vi "RUSHShoot.vi"(1 "In Cluster":T2) -> (0 "Out Cluster":T1)   [LabVIEW 2012]
panel:
  in  "Highest POT pos":dbl=5.0
  in  "Lowest POT pos":dbl
  in  "ShootPOTToPowConst":dbl=0.2
  in  "Vision Speed Const":dbl=0.75
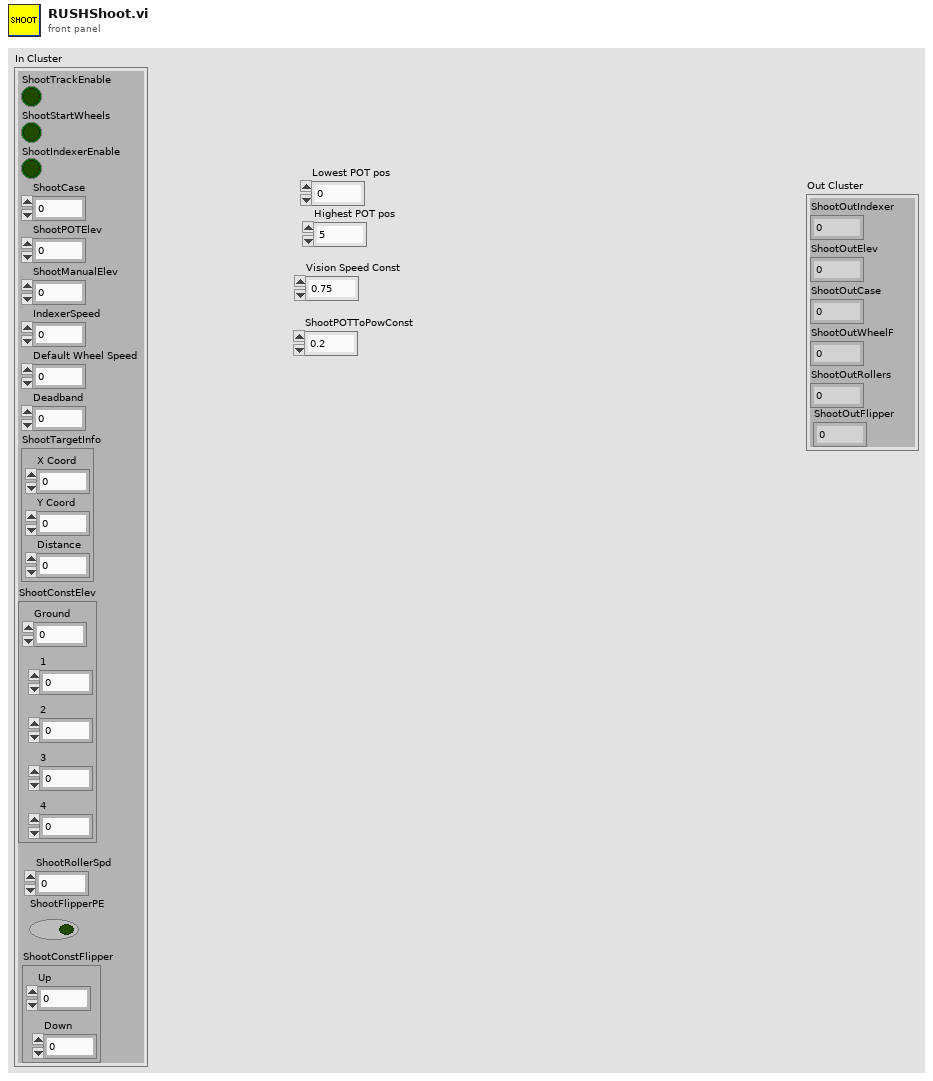
[diagram p1: front panel]
types:
  T1 = cluster{"ShootOutIndexer":dbl, "ShootOutElev":dbl, "ShootOutCase":dbl, "ShootOutWheelF":dbl, "ShootOutRollers":dbl, "ShootOutFlipper":dbl}
  T2 = cluster{"ShootTrackEnable":bool, "ShootStartWheels":bool, "ShootIndexerEnable":bool, "ShootCase":dbl, "ShootPOTElev":dbl, "ShootManualElev":dbl, "IndexerSpeed":dbl, "Default Wheel Speed":dbl, "Deadband":dbl, "ShootTargetInfo":cluster{"X Coord":dbl, "Y Coord":dbl, "Distance":dbl}, "ShootConstElev":cluster{"1":dbl, "2":dbl, "3":dbl, "4":dbl, "Ground":dbl}, "ShootRollerSpd":dbl, "ShootFlipperPE":bool, "ShootConstFlipper":cluster{"Down":dbl, "Up":dbl}}
  T3 = cluster{"X Coord":dbl, "Y Coord":dbl, "Distance":dbl}
  T4 = cluster{"1":dbl, "2":dbl, "3":dbl, "4":dbl, "Ground":dbl}
  T5 = cluster{"f":dbl, "y":dbl, "f":dbl, "f":dbl, "f":dbl, "Down":dbl}
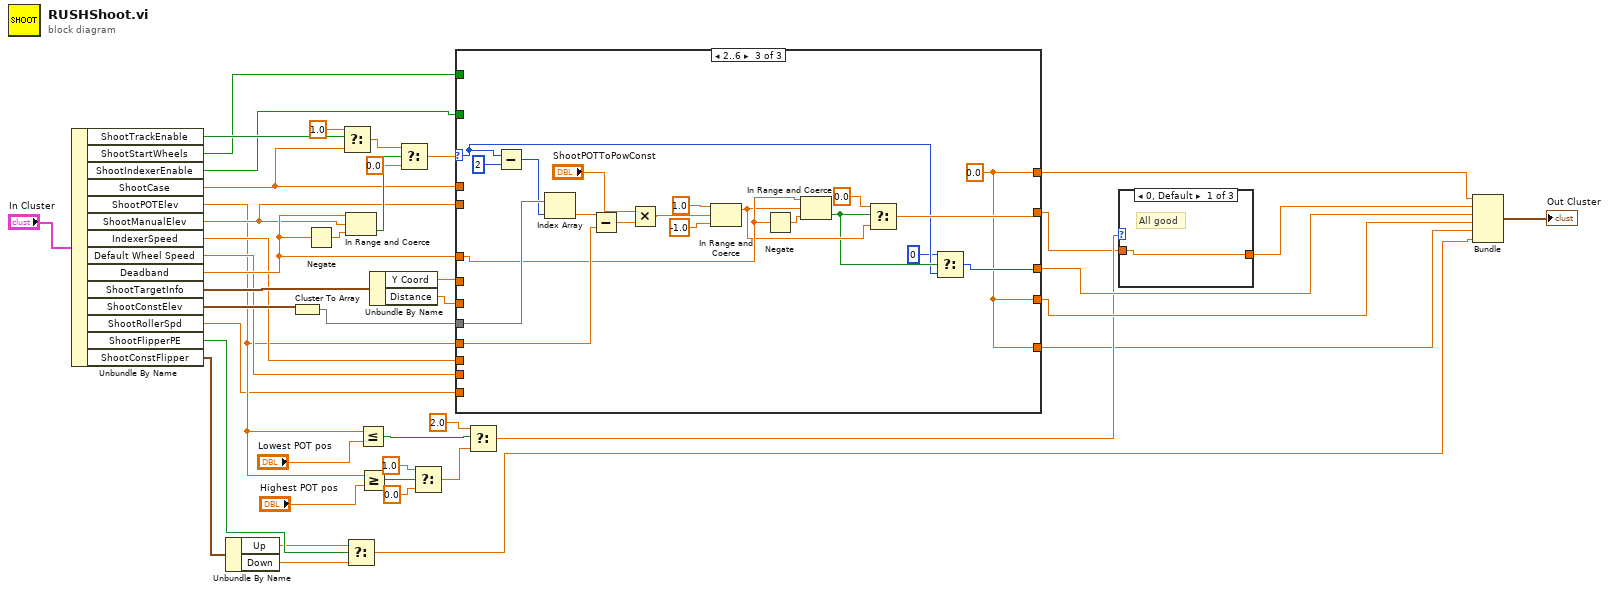
[diagram p0: block diagram]
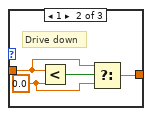
[diagram p2: hidden frame]
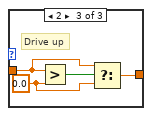
[diagram p3: hidden frame]
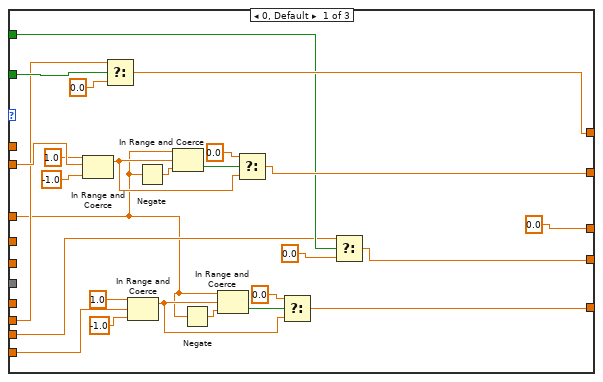
[diagram p4: hidden frame]
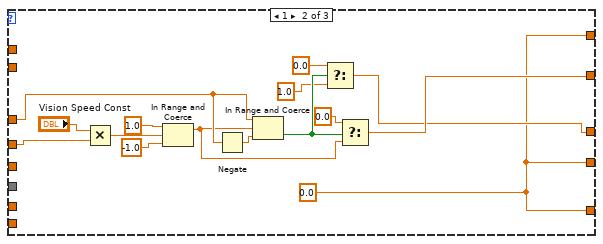
[diagram p5: hidden frame]
diagram:
  n1 = Unbundle By Name("In Cluster") -> ("ShootTrackEnable"=w42:bool, "ShootStartWheels"=w30:bool, "ShootIndexerEnable"=w29:bool, "ShootCase"=w31:dbl, "ShootPOTElev"=w18:dbl, "ShootManualElev"=w28:dbl, "IndexerSpeed"=w21:dbl, "Default Wheel Speed"=w20:dbl, "Deadband"=w32:dbl, "ShootTargetInfo"=w35:T3, "ShootConstElev"=w27:T4, "ShootRollerSpd"=w7:dbl, "ShootFlipperPE"=w3:bool, "ShootConstFlipper"=w4:cluster{"Down":dbl, "Up":dbl})
  n2 = Unbundle By Name(w4) -> ("Up"=w2:dbl, "Down"=w5:dbl)
  n3 = Cluster To Array(cluster=w27) -> (array=w26:dbl[])
  n4 = Negate(x=w32) -> (-x=w39:dbl)
  n5 = Select(t=1.0, s=w42, f=w31) -> (s? t:f=w40:dbl)
  n6 = In Range and Coerce(upper limit=w32, x=w28, lower limit=w39) -> (In Range?=w38:bool)  [unwired: 1 out]
  n7 = Select(t=w2, s=w3, f=w5) -> (s? t:f=w1:dbl)
  n8 = Less Or Equal?(x=w18, y="Lowest POT pos") -> (x <= y?=w12:bool)
  n9 = Greater Or Equal?(x=w18, y="Highest POT pos") -> (x >= y?=w16:bool)
  n10 = Unbundle By Name(w35) -> ("Y Coord"=w34:dbl, "Distance"=w33:dbl)
  n11 = Select(t=w40, s=w38, f=0.0) -> (s? t:f=w36:dbl)
  n12 = Select(t=1.0, s=w16, f=0.0) -> (s? t:f=w13:dbl)
  n13 = case shown="2..6" w36 {
    selector: w36 -> [_ _ w88]
    tunnel: w34 -> [_ w83 _]
    tunnel: w33 -> [_ _ _]
    tunnel: w32 -> [w45 w78 w93]
    tunnel: [0.0 ("upper limit") w72 w86] -> w24
    tunnel: w31 -> [_ _ _]
    tunnel: [w60 w73 w90] -> w9
    tunnel: [w57 w70 w85] -> w23
    tunnel: [w67 w70 w85] -> w25
    tunnel: w30 -> [w58 _ _]
    tunnel: w29 -> [w69 _ _]
    tunnel: w28 -> [w64 _ _]
    tunnel: w26 -> [_ _ w103]
    tunnel: w18 -> [_ _ w100]
    tunnel: w21 -> [w53 _ _]
    tunnel: w20 -> [w54 _ _]
    tunnel: w7 -> [w46 _ _]
    tunnel: [w44 w70 w85] -> w6
    frame 0, Default {
      n14 = In Range and Coerce(upper limit=1.0, x=w64, lower limit=-1.0 ("upper limit")) -> (coerced(x)=w61:dbl)  [unwired: 1 out]
      n15 = Select(t=w53, s=w69, f=0.0) -> (s? t:f=w67:dbl)
      n16 = In Range and Coerce(upper limit=1.0, x=w46, lower limit=-1.0 ("upper limit")) -> (coerced(x)=w51:dbl)  [unwired: 1 out]
      n17 = Negate(x=w45) -> (-x=w65:dbl)
      n18 = In Range and Coerce(upper limit=w45, x=w61, lower limit=w65) -> (In Range?=w63:bool)  [unwired: 1 out]
      n19 = Negate(x=w45) -> (-x=w48:dbl)
      n20 = In Range and Coerce(upper limit=w45, x=w51, lower limit=w48) -> (In Range?=w49:bool)  [unwired: 1 out]
      n21 = Select(t=0.0, s=w63, f=w61) -> (s? t:f=w60:dbl)
      n22 = Select(t=0.0, s=w49, f=w51) -> (s? t:f=w44:dbl)
      n23 = Select(t=w54, s=w58, f=0.0 ("t")) -> (s? t:f=w57:dbl)
    }
    frame 1 {
      w70 = 0.0
      n24 = Multiply(x="Vision Speed Const", y=w83) -> (x*y=w82:dbl)
      n25 = In Range and Coerce(upper limit=1.0, x=w82, lower limit=-1.0 ("upper limit")) -> (coerced(x)=w76:dbl)  [unwired: 1 out]
      n26 = Negate(x=w78) -> (-x=w79:dbl)
      n27 = In Range and Coerce(upper limit=w78, x=w76, lower limit=w79) -> (In Range?=w75:bool)  [unwired: 1 out]
      n28 = Select(t=0.0, s=w75, f=1.0) -> (s? t:f=w72:dbl)
      n29 = Select(t=0.0, s=w75, f=w76) -> (s? t:f=w73:dbl)
    }
    frame 2..6 {
      w85 = 0.0 ("f")
      n30 = Subtract(x=w88, y=2) -> (x-y=w102:i32)
      n31 = Index Array(array=w103, index=w102) -> (element=w101:dbl)
      n32 = Subtract(x=w101, y=w100) -> (x-y=w99:dbl)
      n33 = Multiply(x="ShootPOTToPowConst", y=w99) -> (x*y=w94:dbl)
      n34 = In Range and Coerce(upper limit=1.0, x=w94, lower limit=-1.0 ("upper limit")) -> (coerced(x)=w91:dbl)  [unwired: 1 out]
      n35 = Negate(x=w93) -> (-x=w95:dbl)
      n36 = In Range and Coerce(upper limit=w93, x=w91, lower limit=w95) -> (In Range?=w89:bool)  [unwired: 1 out]
      n37 = Select(t=0.0, s=w89, f=w91) -> (s? t:f=w90:dbl)
      n38 = Select(t=0, s=w89, f=w88) -> (s? t:f=w86:i32)
    }
  }
  n39 = Select(t=2.0, s=w12, f=w13) -> (s? t:f=w10:dbl)
  n40 = case shown="0, Default" w10 {
    tunnel: w9 -> [w105 w107 w111]
    tunnel: [w105 w106 w110] -> w8
    frame 0, Default {
      # "All good"
    }
    frame 1 {
      w108 = 0.0 ("y")
      # "Drive down"
      n41 = Less?(x=w107, y=w108) -> (x < y?=w109:bool)
      n42 = Select(t=w107, s=w109, f=w108) -> (s? t:f=w106:dbl)
    }
    frame 2 {
      w112 = 0.0 ("y")
      # "Drive up"
      n43 = Greater?(x=w111, y=w112) -> (0:w113:bool)
      n44 = Select(t=w111, s=w113, f=w112) -> (s? t:f=w110:dbl)
    }
  }
  n45 = Bundle("f"=w25, "y"=w8, "f"=w24, "f"=w23, "f"=w6, "Down"=w1) -> (→"Out Cluster":T5)  [unwired: 1 in]
